vi "Stamp 3 interface.vi"(6 "Stamp Command":T6, 7 "stamp timeout":i16=5, 8 "error in (no error)":errorcluster, 10 "Control":T1 {"Pumps"."0 to 1" format="%.2f"; "Pumps"."flow rate" format="%.2f"}, 11 "Serial Port":refnum<visa-resource-name>) -> (0 "error out":errorcluster, 1 "success?":bool, 4 "tries":i32)   [LabVIEW 2010]
uses:
  stamp command.ctl
  Stamp 2 control.ctl
  Peristaltic/Pump w direction.ctl
  mini peristaltic pump.ctl
  Pump Direction.ctl
  3-stop colors and numbers.ctl
  <vilib>/Instr/_visa.llb/VISA Configure Serial Port (Instr).vi
panel:
  out "command string":string[](array[string])
  out "responses":string[](array[string])
  out "first subarray":bool[](array[boolean])
  out "second subarray":bool[](array[boolean])
  # "pump2"
  # "0-12"
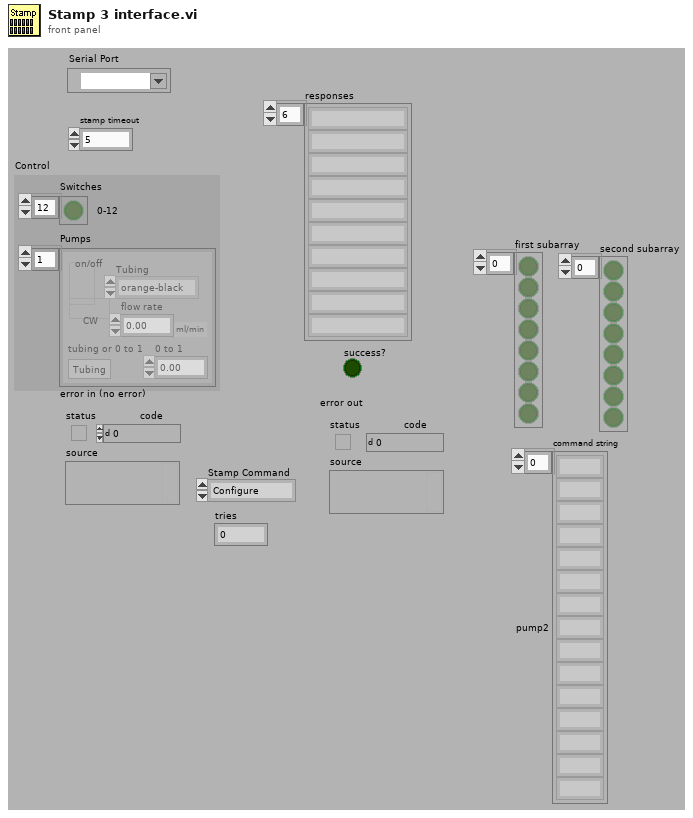
[diagram p1: front panel]
types:
  T1 = typedef "Stamp 2 control.ctl" = cluster{"Switches":bool[], "Pumps":T2[]}
  T2 = typedef "Pump w direction.ctl" = cluster{"on/off":T3, "Direction":T4, "flow rate":dbl[unit], "Tubing":T5, "tubing or 0 to 1":bool, "0 to 1":dbl}
  T3 = typedef "mini peristaltic pump.ctl" = bool
  T4 = typedef "Pump Direction.ctl" = bool
  T5 = typedef "3-stop colors and numbers.ctl" = enum16{"orange-black", "orange-red", "orange-blue", "orange-green", "green-yellow", "orange-yellow", "white-yellow", "orange-white", "black-black", "orange-orange", "white-black", "white-white", "white-red", "red-red", "red-grey", "grey-grey", "yellow-yellow", "yellow-blue", "blue-blue", "blue-green", "green-green", "purple-purple", "purple-black", "purple-orange", "purple-white", "black-white", "13", "14", "15", "16", "17", "18"}
  T6 = typedef "stamp command.ctl" = enum16{"Configure", "Write", "Off", "Close"}
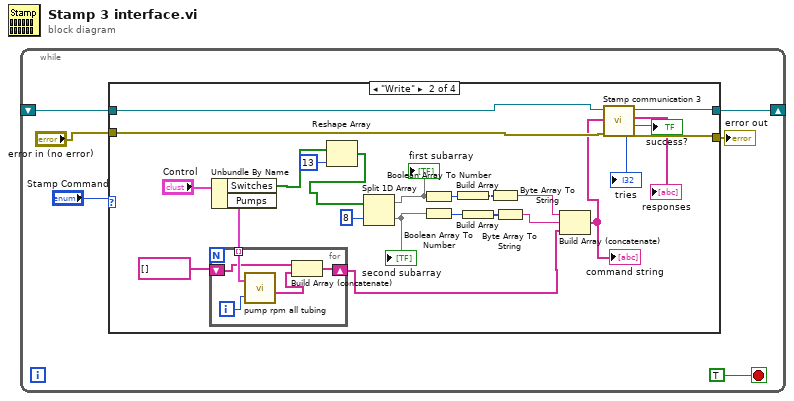
[diagram p0: block diagram]
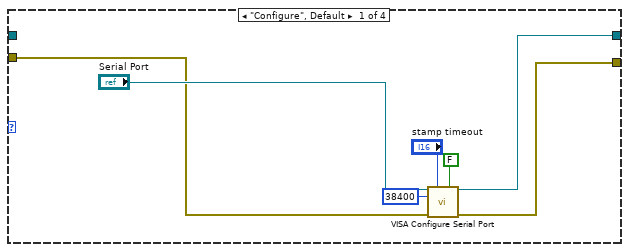
[diagram p2: hidden frame]
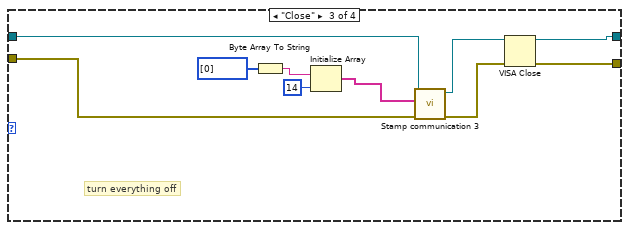
[diagram p3: hidden frame]
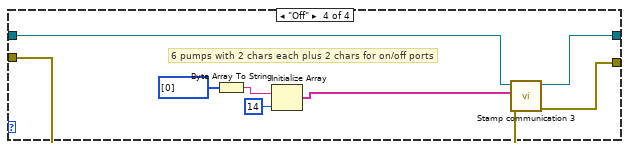
[diagram p4: hidden frame]
diagram:
  n1 = while {
    shift-right: [w2] -> _
    shift-left: _ -> [w1]
    stop <- TRUE stop-if-true
    n2 = case shown="\"Write\"" "Stamp Command" {
      tunnel: "error in (no error)" -> [w12 w29 w48 w57]
      tunnel: [w11 w26 w51 w56] -> w3
      tunnel: [w10 w27 w49 w58] -> w2
      tunnel: w1 -> [_ w28 w50 w59]
      frame "Configure", Default {
        n3 = call-poly "VISA Configure Serial Port"("VISA resource name"="Serial Port", "timeout (10sec)"="stamp timeout", "Enable Termination\nChar (T)"=FALSE ("Enable Termination\nChar (T)"), "baud rate (9600)"=u32 38400, "error in (no error)"=w12) -> ("VISA resource name out"=w10:refnum<visa-resource-name>, "error out"=w11:errorcluster)  [unwired: 9 in]
      }
      frame "Write" {
        n4 = Unbundle By Name("Control") -> ("Switches"=w32:bool[], "Pumps"=w36:T2[])
        n5 = for {
          tunnel: w36 -> [w42] mode=indexing
          shift-right: [w40] -> w18
          shift-left: string[] [] ("command chars") -> [w39]
          i -> [w38]
          n6 = call "pump rpm all tubing.vi"("Pump"=w42, "pump ID"=w38) -> ("command chars"=w41:string[])  [unwired: 3 out]
          n7 = Build Array (concatenate)(w39, w41) -> (w40:string[])
        }
        n8 = Reshape Array(w32, 13 ("dimension size")) -> (w22:bool[])
        n9 = Split 1D Array(array=w22, index=8 ("length")) -> (first subarray=w34:bool[], second subarray=w33:bool[])
        "second subarray" <- w33
        "first subarray" <- w34
        n10 = Boolean Array To Number(Boolean array=w34) -> (number=w30:u32)
        n11 = Boolean Array To Number(Boolean array=w33) -> (number=w15:u32)
        n12 = Build Array(w30) -> (w21:u32[])
        n13 = Build Array(w15) -> (w16:u32[])
        n14 = Byte Array To String(unsigned byte array=w21) -> (string=w17:string)
        n15 = Byte Array To String(unsigned byte array=w16) -> (string=w14:string)
        n16 = Build Array (concatenate)(w17, w14, w18) -> (w20:string[])
        "command string" <- w20
        n17 = call "Stamp communication 3.vi"("error in (no error)"=w29, "command array"=w20, "Serial Port"=w28) -> ("error out"=w26:errorcluster, "Success"=→"success?":bool, "responses"=→"responses":string[], "Serial Port out"=w27:refnum<visa-resource-name>, "tries"=→"tries":i32)  [unwired: 3 in, 1 out]
      }
      frame "Close" {
        # "turn everything off"
        n18 = Byte Array To String(unsigned byte array=u8[] [0]) -> (string=w45:string)
        n19 = Initialize Array(w45, 14 ("dimension size")) -> (w43:string[])
        n20 = call "Stamp communication 3.vi"("error in (no error)"=w48, "command array"=w43, "Serial Port"=w50) -> ("error out"=w47:errorcluster, "Serial Port out"=w49:refnum<visa-resource-name>)  [unwired: 3 in, 4 out]
        n21 = VISA Close(VISA resource name=w49, error in (no error)=w47) -> (error out=w51:errorcluster)
      }
      frame "Off" {
        # "6 pumps with 2 chars each plus 2 chars for on/off ports"
        n22 = Byte Array To String(unsigned byte array=u8[] [0]) -> (string=w54:string)
        n23 = Initialize Array(w54, 14 ("dimension size")) -> (w52:string[])
        n24 = call "Stamp communication 3.vi"("error in (no error)"=w57, "command array"=w52, "Serial Port"=w59) -> ("error out"=w56:errorcluster, "Serial Port out"=w58:refnum<visa-resource-name>)  [unwired: 3 in, 4 out]
      }
    }
    "error out" <- w3
  }
